vi "Setup Motors.vi"   [LabVIEW 2014]
uses:
  <vilib>/Rock Robotics/SystemInterfaces/DIO/FPGA_DIOPWMChannel.ctl
  <vilib>/Rock Robotics/WPI/Joystick/WPI_JoystickDeviceEnum.ctl
  <vilib>/Rock Robotics/SystemInterfaces/Typedef/FPGA_TypedefAnalogModule.ctl
  <vilib>/Rock Robotics/SystemInterfaces/AI/FPGA_AIChannel.ctl
  <vilib>/Rock Robotics/SystemInterfaces/Typedef/FPGA_TypedefDigitalModule.ctl
  <vilib>/Rock Robotics/WPI/Solenoid/WPI_SolenoidChannel.ctl
  <vilib>/Rock Robotics/SystemInterfaces/AI/FPGA_AIGyroChannel.ctl
  <vilib>/Rock Robotics/SystemInterfaces/Typedef/FPGA_TypedefAnalogModuleForGyro.ctl
  <vilib>/Rock Robotics/SystemInterfaces/DIO/FPGA_DIOChannel.ctl
  <vilib>/Rock Robotics/WPI/SafetyOutput/WPI_SafetyOutputConfigMenu.ctl
  NavX Code/navX-MXP Library/COMMON/TypeDefs/Value TypeDefs/navX Interface Protocol.ctl
  <vilib>/Rock Robotics/SystemInterfaces/spilib/spi_bus.ctl
  <vilib>/Rock Robotics/SystemInterfaces/i2clib/i2c_bus.ctl
  NavX Code/navX-MXP Library/COMMON/TypeDefs/Value TypeDefs/navX Update Rate.ctl
  <vilib>/Rock Robotics/WPI/MotorControl/WPI_MotorControlOpen Jaguar.vi
  <vilib>/Rock Robotics/WPI/MotorControl/WPI_MotorControlOpen Talon.vi
  <vilib>/Rock Robotics/WPI/Solenoid/WPI_SolenoidOpenSingle.vi
  <vilib>/Rock Robotics/WPI/Switch/WPI_SwitchOpenLimit.vi
  <vilib>/Rock Robotics/WPI/Counter/WPI_CounterDigitalInputToDigitalSource.vi
  <vilib>/Rock Robotics/WPI/Counter/WPI_CounterOpen UpDown Mode.vi
  Global Variables.vi
  NavX Code/navX-MXP Library/navX-MXP IMU.lvlib
types:
  T1 = typedef "navX-MXP IMU.lvlib/navX Update Rate.ctl" = u8
  T2 = typedef "i2c_bus.ctl" = enum16{"I2C On-Board", "I2C MXP", "Invalid"}
  T3 = typedef "spi_bus.ctl" = enum16{"SPI On-Board, CS0", "SPI On-Board, CS1", "SPI On-Board, CS2", "SPI On-Board, CS3", "SPI MXP", "Invalid"}
  T4 = typedef "navX-MXP IMU.lvlib/navX Interface Protocol.ctl" = enum16{"SPI", "I2C"}
  T5 = typedef "FPGA_DIOChannel.ctl" = enum8{"DIO 0", "DIO 1", "DIO 2", "DIO 3", "DIO 4", "DIO 5", "DIO 6", "DIO 7", "DIO 8", "DIO 9", "DIO MXP 0", "DIO MXP 1", "DIO MXP 2", "DIO MXP 3", "DIO MXP 4", "DIO MXP 5", "DIO MXP 6", "DIO MXP 7", "DIO MXP 8", "DIO MXP 9", "DIO MXP 10", "DIO MXP 11", "DIO MXP 12", "DIO MXP 13", "DIO MXP 14", "DIO MXP 15", "Invalid"}
  T6 = typedef "WPI_SafetyOutputConfigMenu.ctl" = enum16{"Enable", "Disable"}
  T7 = typedef "FPGA_TypedefDigitalModule.ctl" = enum16{"Controller 1"}
  T8 = typedef "FPGA_TypedefAnalogModuleForGyro.ctl" = enum16{"Controller 1"}
  T9 = typedef "FPGA_AIGyroChannel.ctl" = enum8{"AI 0", "AI 1", "Invalid"}
  T10 = typedef "WPI_SolenoidChannel.ctl" = enum8{"Solenoid 0", "Solenoid 1", "Solenoid 2", "Solenoid 3", "Solenoid 4", "Solenoid 5", "Solenoid 6", "Solenoid 7", "Invalid"}
  T11 = typedef "FPGA_DIOPWMChannel.ctl" = enum8{"PWM 0", "PWM 1", "PWM 2", "PWM 3", "PWM 4", "PWM 5", "PWM 6", "PWM 7", "PWM 8", "PWM 9", "PWM MXP 0", "PWM MXP 1", "PWM MXP 2", "PWM MXP 3", "PWM MXP 4", "PWM MXP 5", "PWM MXP 6", "PWM MXP 7", "PWM MXP 8", "PWM MXP 9", "Invalid"}
  T12 = typedef "FPGA_AIChannel.ctl" = enum8{"AI 0", "AI 1", "AI 2", "AI 3", "AI MXP 0", "AI MXP 1", "AI MXP 2", "AI MXP 3", "Invalid"}
  T13 = typedef "FPGA_TypedefAnalogModule.ctl" = enum16{"Controller 1"}
  T14 = typedef "WPI_JoystickDeviceEnum.ctl" = enum16{"USB 0", "USB 1", "USB 2", "USB 3", "USB 4", "USB 5"}
  T15 = typedef "WPI_MotorControlDeviceRef.ctl" = cluster{"DeviceStatus":errorcluster, "Type":T16, "PWM":cluster{"Controller":T7, "PWM Channel":T11, "DeadBand":T17}, "CAN":cluster{"Device Number":u8, "Control Mode":T18, "Semaphore":T19, "Max Vout":dbl, "TalonSRX Control Mode":T20}, "Invert":bool, "TransformRef":T21, "InvTransformRef":T21}
  T16 = typedef "WPI_MotorControlType.ctl" = enum16{"PWM", "CAN", "CANTalonSRX"}
  T17 = typedef "WPI_PWMDeadband.ctl" = cluster{"Name":string, "maxPositivePwm":i32, "minPositivePwm":i32, "centerPwm":i32, "maxNegativePwm":i32, "minNegativePwm":i32, "angularRange":u16}
  T18 = typedef "WPI_CANJaguar_ControlMode.ctl" = enum8{"Percent VBus", "Current", "Speed", "Position", "Voltage"}
  T19 = typedef "Semaphore RefNum" = refnum<k1>
  T20 = typedef "WPI_CANTalonSRX_APIControlMode.ctl" = enum8{"Percent VBus", "Speed", "Position", "Slave", "Unchanged / Invalid"}
  T21 = typedef "WPI_PWMTransform_ConPane.ctl" = refnum<vi>
  T22 = typedef "WPI_GyroDevRef.ctl" = cluster{"DevStatus":errorcluster, "Analog Module":T13, "Analog Channel":T12, "Offset":dbl, "Gain (VoltsPerDegree/Second)":dbl}
  T23 = typedef "WPI_SolenoidDevRef.ctl" = cluster{"DevStatus":errorcluster, "Pneumatics Control Module":u8, "Forward Solenoid Channel":T10, "Reverse Solenoid Channel":T10}
  T24 = typedef "WPI_SwitchDevRef.ctl" = cluster{"DevStatus":errorcluster, "DIO Channel":T5, "Controller":T7, "CntIndex":T25, "Normally Closed":bool}
  T25 = typedef "FPGA_CounterCtrSystemIndex.ctl" = enum8{"Ctr 0", "Ctr 1", "Ctr 2", "Ctr 3", "Ctr 4", "Ctr 5", "Ctr 6", "Ctr 7", "Invalid"}
  T26 = typedef "WPI_AnalogChannelDevRef.ctl" = cluster{"DevStatus":errorcluster, "Controller":T13, "Analog Channel":T12}
  T27 = typedef "WPI_DigitalInputDevRef.ctl" = cluster{"DevStatus":errorcluster, "DIO Channel":T5, "Controller":T7}
  T28 = typedef "FPGA_CounterEncoderSourceConvertionLVSourceType.ctl" = cluster{"DevStatus":errorcluster, "AnalogTriggerMode?":bool, "DigitalMode":cluster{"Controller":T7, "DIO Channel":T29}, "AnalogTriggerMode":cluster{"AnalogTriggerIndex":T30, "OutputType":T31}}
  T29 = typedef "FPGA_DIODigitalSourceChannel.ctl" = enum8{"DIO 0", "DIO 1", "DIO 2", "DIO 3", "DIO 4", "DIO 5", "DIO 6", "DIO 7", "DIO 8", "DIO 9", "DIO MXP 0", "DIO MXP 1", "DIO MXP 2", "DIO MXP 3", "DIO MXP 4", "DIO MXP 5", "DIO MXP 6", "DIO MXP 7", "DIO MXP 8", "DIO MXP 9", "DIO MXP 10", "DIO MXP 11", "DIO MXP 12", "DIO MXP 13", "DIO MXP 14", "DIO MXP 15", "Disabled"}
  T30 = typedef "FPGA_AnalogTriggerIndex.ctl" = enum8{"Trig 0", "Trig 1", "Trig 2", "Trig 3", "Trig 4", "Trig 5", "Trig 6", "Trig 7", "Invalid"}
  T31 = typedef "FPGA_AnalogTriggerOutType.ctl" = enum16{"InWindow", "TriggerState", "Rising", "Falling"}
  T32 = typedef "WPI_EncoderDevRef.ctl" = cluster{"DevStatus":errorcluster, "EncoderIndex":T33, "CounterIndex":T25, "DistancePerCount":dbl, "Decoding Type":T34}
  T33 = typedef "FPGA_EncoderIdx.ctl" = enum8{"Enc 0", "Enc 1", "Enc 2", "Enc 3", "Enc 4", "Enc 5", "Enc 6", "Enc 7", "Invalid"}
  T34 = typedef "WPI_EncoderType.ctl" = enum16{"1x", "2x", "4x"}
  T35 = typedef "WPI_CounterDevRef.ctl" = cluster{"DevStatus":errorcluster, "CntIndex":T25}
  T36 = typedef "navX-MXP IMU.lvlib/navX Device TypeDef.ctl" = cluster{"navX Interface Protocol":T4, "navX Interface Protocol TypeDefs":cluster{"SPIDevRef":T37, "I2CDevRef":T38}, "navX System Information":cluster{"Board Information":T39, "Status":T40, "Offsets":T44}, "navX Common Information":cluster{"Update Rate (4Hz-60Hz)":T1, "refnum name":string, "error":errorcluster}}
  T37 = typedef "WPI_SPIDevRef.ctl" = cluster{"DevStatus":errorcluster, "Handle":i32, "Controller":T7, "SPI Bus":T3}
  T38 = typedef "WPI_I2CDevRef.ctl" = cluster{"DevStatus":errorcluster, "Controller":T7, "Device Address":u8, "Handle":i32, "I2C Bus":T2}
  T39 = typedef "navX-MXP IMU.lvlib/navX Board Information.ctl" = cluster{"WhoAmI (50 | 0x32)":u8, "Board Revision":u8, "Firmware Major Version":u8, "Firmware Minor Version":u8}
  T40 = typedef "navX-MXP IMU.lvlib/navX Status Data.ctl" = cluster{"Update Rate Hz":u8, "Accelerometer Full-Scale Range":u8, "Gyro Full-Scale Range":u16, "NAVX_OP_STATUS":T41, "NAVX_CAL_STATUS":T42, "NAVX_SELFTEST_STATUS":u8, "NAVX_SENSOR_STATUS":T43}
  T41 = typedef "navX-MXP IMU.lvlib/navX NAVX_OP_STATUS.ctl" = u8
  T42 = typedef "navX-MXP IMU.lvlib/navX NAVX_CAL_STATUS.ctl" = u8
  T43 = typedef "navX-MXP IMU.lvlib/navX NAVX_SENSOR_STATUS.ctl" = cluster{"MOVING":bool, "YAW_STABLE":bool, "MAG_DISTURBANCE":bool, "ALTITUDE_VALID":bool, "SEALEVEL_PRESS_SET":bool, "FUSED_HEADING_VALID":bool}
  T44 = typedef "navX-MXP IMU.lvlib/navX Offsets Data.ctl" = cluster{"Yaw":dbl, "Quat W":dbl, "Quat X":dbl, "Quat Y":dbl, "Quat Z":dbl}
  T45 = typedef "WPI_JoystickDevRef.ctl" = cluster{"Device":T14}
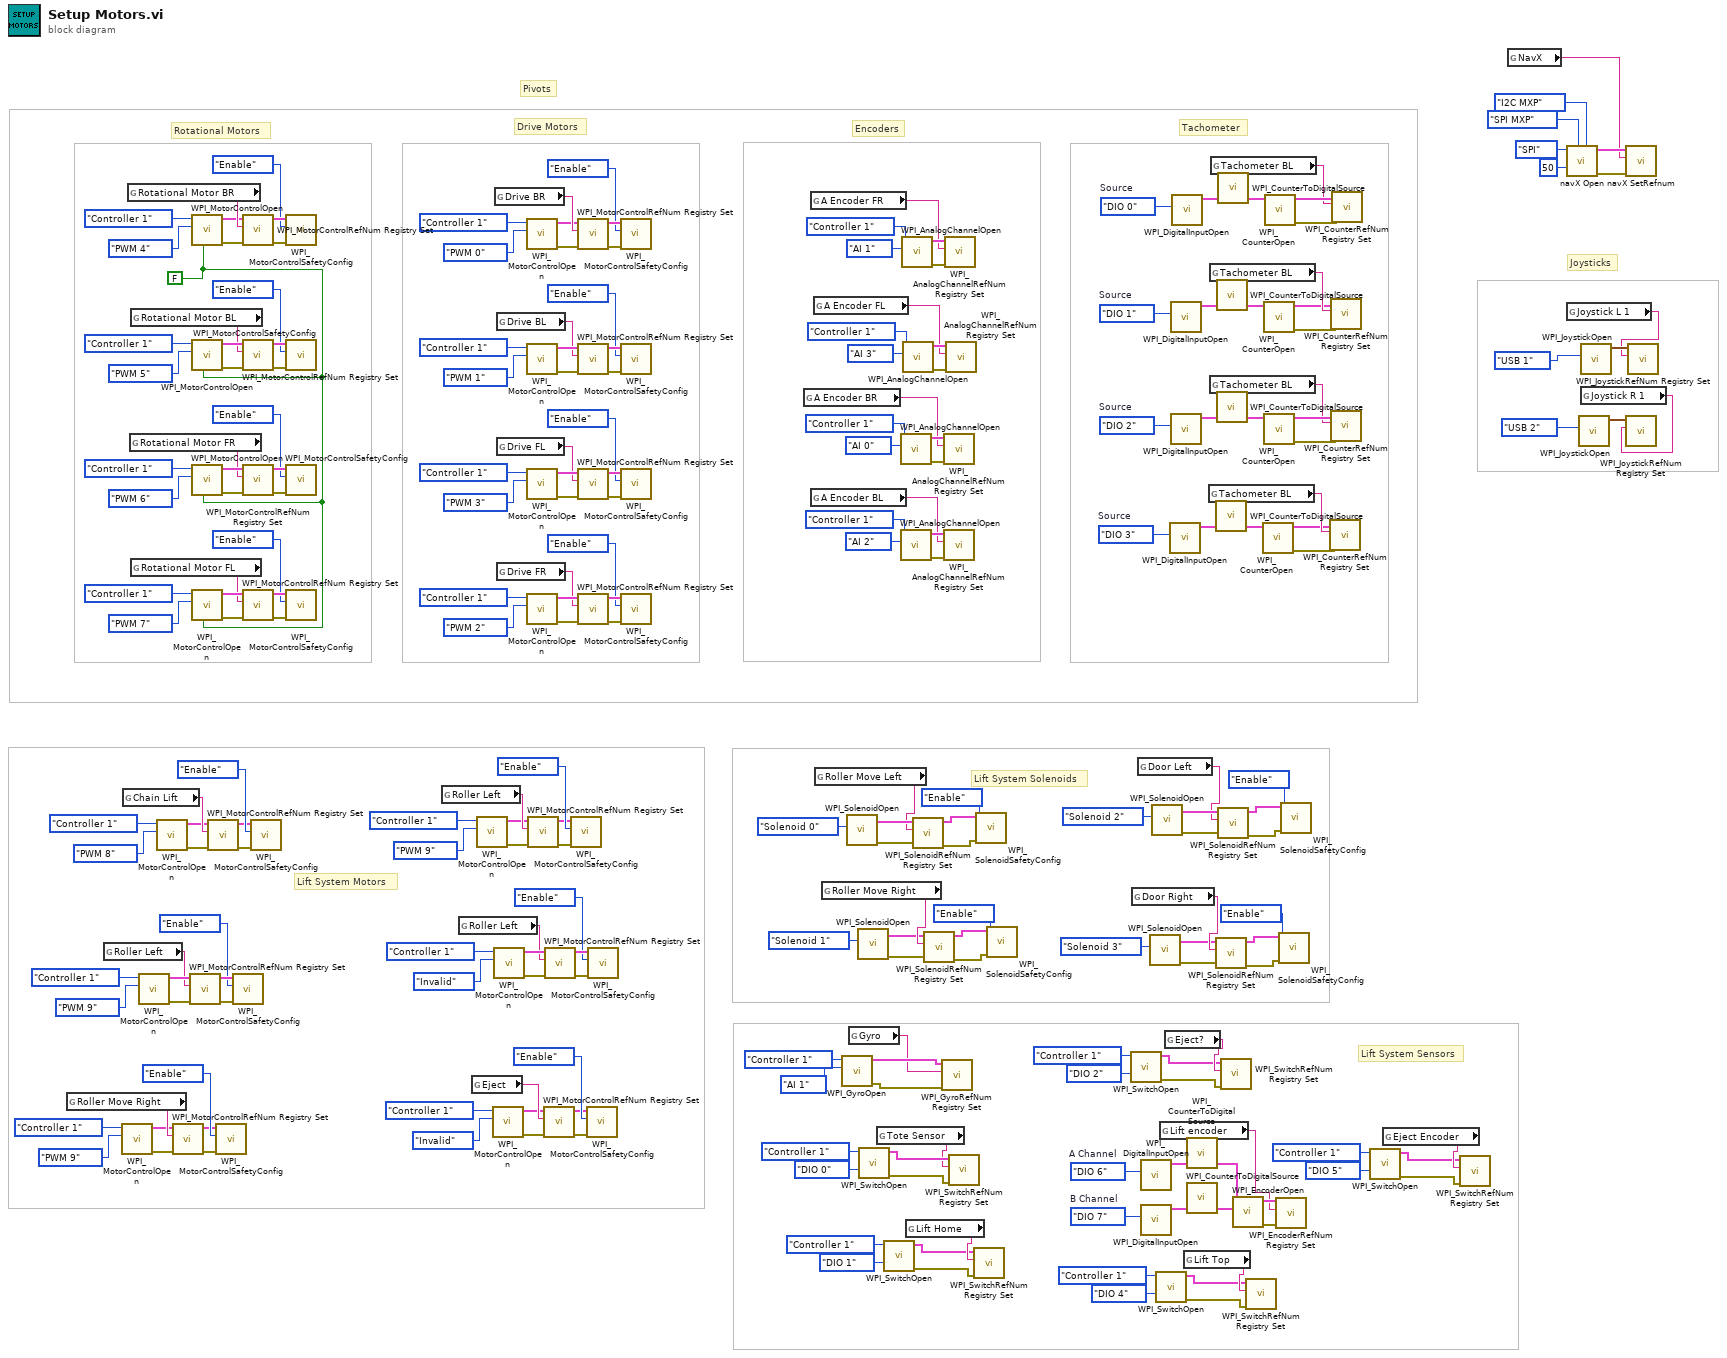
[diagram p0: block diagram]
diagram:
  w9 = FPGA_DIOChannel."DIO 3"  # Source
  w18 = FPGA_DIOChannel."DIO 2"  # Source
  w21 = FPGA_DIOChannel."DIO 1"  # Source
  w30 = FPGA_DIOChannel."DIO 0"  # Source
  w32 = FALSE ("Invert")
  w41 = FPGA_DIOChannel."DIO 7"  # B Channel
  w40 = FPGA_DIOChannel."DIO 6"  # A Channel
  # "Tachometer"
  # "Lift System Sensors"
  # "Lift System Solenoids"
  # "Lift System Motors"
  # "Encoders"
  # "Joysticks"
  # "Pivots"
  # "Rotational Motors"
  # "Drive Motors"
  n1 = global read "Global Variables.vi" "Roller Move Right"() -> (w130:string)
  n2 = global read "Global Variables.vi" "Roller Left"() -> (w133:string)
  n3 = call-poly <vilib>:"WPI_MotorControlOpen.vi"("PWM Channel"=FPGA_DIOPWMChannel."PWM 9", "Controller"=FPGA_TypedefDigitalModule."Controller 1") -> ("error out"=w125:errorcluster, "MotorControlDeviceRef"=w124:T15)  [unwired: 8 in]
  n4 = global read "Global Variables.vi" "Chain Lift"() -> (w146:string)
  n5 = global read "Global Variables.vi" "Rotational Motor BR"() -> (w200:string)
  n6 = global read "Global Variables.vi" "Rotational Motor FR"() -> (w174:string)
  n7 = global read "Global Variables.vi" "Rotational Motor BL"() -> (w175:string)
  n8 = global read "Global Variables.vi" "Rotational Motor FL"() -> (w173:string)
  n9 = call-poly <vilib>:"WPI_MotorControlOpen.vi"("PWM Channel"=FPGA_DIOPWMChannel."PWM 9", "Controller"=FPGA_TypedefDigitalModule."Controller 1") -> ("error out"=w138:errorcluster, "MotorControlDeviceRef"=w139:T15)  [unwired: 8 in]
  n10 = call-poly <vilib>:"WPI_MotorControlOpen.vi"("PWM Channel"=FPGA_DIOPWMChannel."PWM 8", "Controller"=FPGA_TypedefDigitalModule."Controller 1") -> ("error out"=w141:errorcluster, "MotorControlDeviceRef"=w140:T15)  [unwired: 8 in]
  n11 = call <vilib>:"WPI_MotorControlRefNum Registry Set.vi"("error in (no error)"=w125, "refnum name"=w130, "MotorControlDevRef"=w124) -> ("error out"=w127:errorcluster, "MotorControlDevRef"=w126:T15)  [unwired: 7 in]
  n12 = call <vilib>:"WPI_MotorControlRefNum Registry Set.vi"("error in (no error)"=w138, "refnum name"=w133, "MotorControlDevRef"=w139) -> ("error out"=w136:errorcluster, "MotorControlDevRef"=w137:T15)  [unwired: 7 in]
  n13 = call-poly <vilib>:"WPI_MotorControlOpen.vi"("Invert"=w32, "PWM Channel"=FPGA_DIOPWMChannel."PWM 4", "Controller"=FPGA_TypedefDigitalModule."Controller 1") -> ("error out"=w198:errorcluster, "MotorControlDeviceRef"=w199:T15)  [unwired: 7 in]
  n14 = call-poly <vilib>:"WPI_MotorControlOpen.vi"("Invert"=w32, "PWM Channel"=FPGA_DIOPWMChannel."PWM 5", "Controller"=FPGA_TypedefDigitalModule."Controller 1") -> ("error out"=w192:errorcluster, "MotorControlDeviceRef"=w193:T15)  [unwired: 7 in]
  n15 = call-poly <vilib>:"WPI_MotorControlOpen.vi"("Invert"=w32, "PWM Channel"=FPGA_DIOPWMChannel."PWM 6", "Controller"=FPGA_TypedefDigitalModule."Controller 1") -> ("error out"=w186:errorcluster, "MotorControlDeviceRef"=w187:T15)  [unwired: 7 in]
  n16 = call-poly <vilib>:"WPI_MotorControlOpen.vi"("Invert"=w32, "PWM Channel"=FPGA_DIOPWMChannel."PWM 7", "Controller"=FPGA_TypedefDigitalModule."Controller 1") -> ("error out"=w180:errorcluster, "MotorControlDeviceRef"=w181:T15)  [unwired: 7 in]
  n17 = call <vilib>:"WPI_MotorControlRefNum Registry Set.vi"("error in (no error)"=w141, "refnum name"=w146, "MotorControlDevRef"=w140) -> ("error out"=w143:errorcluster, "MotorControlDevRef"=w142:T15)  [unwired: 7 in]
  n18 = call <vilib>:"WPI_MotorControlSafetyConfig.vi"("error in (no error)"=w127, "mode"=WPI_SafetyOutputConfigMenu."Enable", "MotorControlDevRef"=w126) -> ()  [unwired: 7 in, 2 out]
  n19 = call <vilib>:"WPI_MotorControlSafetyConfig.vi"("error in (no error)"=w136, "mode"=WPI_SafetyOutputConfigMenu."Enable", "MotorControlDevRef"=w137) -> ()  [unwired: 7 in, 2 out]
  n20 = call <vilib>:"WPI_MotorControlRefNum Registry Set.vi"("error in (no error)"=w198, "refnum name"=w200, "MotorControlDevRef"=w199) -> ("error out"=w196:errorcluster, "MotorControlDevRef"=w197:T15)  [unwired: 7 in]
  n21 = call <vilib>:"WPI_MotorControlRefNum Registry Set.vi"("error in (no error)"=w192, "refnum name"=w175, "MotorControlDevRef"=w193) -> ("error out"=w190:errorcluster, "MotorControlDevRef"=w191:T15)  [unwired: 7 in]
  n22 = call <vilib>:"WPI_MotorControlRefNum Registry Set.vi"("error in (no error)"=w186, "refnum name"=w174, "MotorControlDevRef"=w187) -> ("error out"=w184:errorcluster, "MotorControlDevRef"=w185:T15)  [unwired: 7 in]
  n23 = call <vilib>:"WPI_MotorControlRefNum Registry Set.vi"("error in (no error)"=w180, "refnum name"=w173, "MotorControlDevRef"=w181) -> ("error out"=w178:errorcluster, "MotorControlDevRef"=w179:T15)  [unwired: 7 in]
  n24 = call <vilib>:"WPI_MotorControlSafetyConfig.vi"("error in (no error)"=w143, "mode"=WPI_SafetyOutputConfigMenu."Enable", "MotorControlDevRef"=w142) -> ()  [unwired: 7 in, 2 out]
  n25 = call <vilib>:"WPI_MotorControlSafetyConfig.vi"("error in (no error)"=w196, "mode"=WPI_SafetyOutputConfigMenu."Enable", "MotorControlDevRef"=w197) -> ()  [unwired: 7 in, 2 out]
  n26 = call <vilib>:"WPI_MotorControlSafetyConfig.vi"("error in (no error)"=w190, "mode"=WPI_SafetyOutputConfigMenu."Enable", "MotorControlDevRef"=w191) -> ()  [unwired: 7 in, 2 out]
  n27 = call <vilib>:"WPI_MotorControlSafetyConfig.vi"("error in (no error)"=w184, "mode"=WPI_SafetyOutputConfigMenu."Enable", "MotorControlDevRef"=w185) -> ()  [unwired: 7 in, 2 out]
  n28 = call <vilib>:"WPI_MotorControlSafetyConfig.vi"("error in (no error)"=w178, "mode"=WPI_SafetyOutputConfigMenu."Enable", "MotorControlDevRef"=w179) -> ()  [unwired: 7 in, 2 out]
  n29 = global read "Global Variables.vi" "Roller Left"() -> (w122:string)
  n30 = global read "Global Variables.vi" "Roller Left"() -> (w109:string)
  n31 = global read "Global Variables.vi" "Eject"() -> (w106:string)
  n32 = call-poly <vilib>:"WPI_MotorControlOpen.vi"("PWM Channel"=FPGA_DIOPWMChannel."PWM 9", "Controller"=FPGA_TypedefDigitalModule."Controller 1") -> ("error out"=w117:errorcluster, "MotorControlDeviceRef"=w116:T15)  [unwired: 8 in]
  n33 = call-poly <vilib>:"WPI_MotorControlOpen.vi"("PWM Channel"=FPGA_DIOPWMChannel."Invalid", "Controller"=FPGA_TypedefDigitalModule."Controller 1") -> ("error out"=w101:errorcluster, "MotorControlDeviceRef"=w100:T15)  [unwired: 8 in]
  n34 = call-poly <vilib>:"WPI_MotorControlOpen.vi"("PWM Channel"=FPGA_DIOPWMChannel."Invalid", "Controller"=FPGA_TypedefDigitalModule."Controller 1") -> ("error out"=w114:errorcluster, "MotorControlDeviceRef"=w115:T15)  [unwired: 8 in]
  n35 = global read "Global Variables.vi" "Drive BR"() -> (w237:string)
  n36 = global read "Global Variables.vi" "Drive BL"() -> (w212:string)
  n37 = global read "Global Variables.vi" "Drive FL"() -> (w211:string)
  n38 = global read "Global Variables.vi" "Drive FR"() -> (w210:string)
  n39 = call-poly <vilib>:"WPI_MotorControlOpen.vi"("PWM Channel"=FPGA_DIOPWMChannel."PWM 0", "Controller"=FPGA_TypedefDigitalModule."Controller 1") -> ("error out"=w235:errorcluster, "MotorControlDeviceRef"=w236:T15)  [unwired: 8 in]
  n40 = call-poly <vilib>:"WPI_MotorControlOpen.vi"("PWM Channel"=FPGA_DIOPWMChannel."PWM 1", "Controller"=FPGA_TypedefDigitalModule."Controller 1") -> ("error out"=w229:errorcluster, "MotorControlDeviceRef"=w230:T15)  [unwired: 8 in]
  n41 = call-poly <vilib>:"WPI_MotorControlOpen.vi"("PWM Channel"=FPGA_DIOPWMChannel."PWM 3", "Controller"=FPGA_TypedefDigitalModule."Controller 1") -> ("error out"=w223:errorcluster, "MotorControlDeviceRef"=w224:T15)  [unwired: 8 in]
  n42 = call-poly <vilib>:"WPI_MotorControlOpen.vi"("PWM Channel"=FPGA_DIOPWMChannel."PWM 2", "Controller"=FPGA_TypedefDigitalModule."Controller 1") -> ("error out"=w217:errorcluster, "MotorControlDeviceRef"=w218:T15)  [unwired: 8 in]
  n43 = call <vilib>:"WPI_MotorControlRefNum Registry Set.vi"("error in (no error)"=w117, "refnum name"=w122, "MotorControlDevRef"=w116) -> ("error out"=w119:errorcluster, "MotorControlDevRef"=w118:T15)  [unwired: 7 in]
  n44 = call <vilib>:"WPI_MotorControlRefNum Registry Set.vi"("error in (no error)"=w101, "refnum name"=w106, "MotorControlDevRef"=w100) -> ("error out"=w103:errorcluster, "MotorControlDevRef"=w102:T15)  [unwired: 7 in]
  n45 = call <vilib>:"WPI_MotorControlRefNum Registry Set.vi"("error in (no error)"=w114, "refnum name"=w109, "MotorControlDevRef"=w115) -> ("error out"=w112:errorcluster, "MotorControlDevRef"=w113:T15)  [unwired: 7 in]
  n46 = call <vilib>:"WPI_MotorControlSafetyConfig.vi"("error in (no error)"=w119, "mode"=WPI_SafetyOutputConfigMenu."Enable", "MotorControlDevRef"=w118) -> ()  [unwired: 7 in, 2 out]
  n47 = call <vilib>:"WPI_MotorControlRefNum Registry Set.vi"("error in (no error)"=w235, "refnum name"=w237, "MotorControlDevRef"=w236) -> ("error out"=w233:errorcluster, "MotorControlDevRef"=w234:T15)  [unwired: 7 in]
  n48 = call <vilib>:"WPI_MotorControlRefNum Registry Set.vi"("error in (no error)"=w229, "refnum name"=w212, "MotorControlDevRef"=w230) -> ("error out"=w227:errorcluster, "MotorControlDevRef"=w228:T15)  [unwired: 7 in]
  n49 = call <vilib>:"WPI_MotorControlRefNum Registry Set.vi"("error in (no error)"=w223, "refnum name"=w211, "MotorControlDevRef"=w224) -> ("error out"=w221:errorcluster, "MotorControlDevRef"=w222:T15)  [unwired: 7 in]
  n50 = call <vilib>:"WPI_MotorControlRefNum Registry Set.vi"("error in (no error)"=w217, "refnum name"=w210, "MotorControlDevRef"=w218) -> ("error out"=w215:errorcluster, "MotorControlDevRef"=w216:T15)  [unwired: 7 in]
  n51 = call <vilib>:"WPI_MotorControlSafetyConfig.vi"("error in (no error)"=w103, "mode"=WPI_SafetyOutputConfigMenu."Enable", "MotorControlDevRef"=w102) -> ()  [unwired: 7 in, 2 out]
  n52 = call <vilib>:"WPI_MotorControlSafetyConfig.vi"("error in (no error)"=w112, "mode"=WPI_SafetyOutputConfigMenu."Enable", "MotorControlDevRef"=w113) -> ()  [unwired: 7 in, 2 out]
  n53 = call <vilib>:"WPI_MotorControlSafetyConfig.vi"("error in (no error)"=w233, "mode"=WPI_SafetyOutputConfigMenu."Enable", "MotorControlDevRef"=w234) -> ()  [unwired: 7 in, 2 out]
  n54 = call <vilib>:"WPI_MotorControlSafetyConfig.vi"("error in (no error)"=w227, "mode"=WPI_SafetyOutputConfigMenu."Enable", "MotorControlDevRef"=w228) -> ()  [unwired: 7 in, 2 out]
  n55 = call <vilib>:"WPI_MotorControlSafetyConfig.vi"("error in (no error)"=w221, "mode"=WPI_SafetyOutputConfigMenu."Enable", "MotorControlDevRef"=w222) -> ()  [unwired: 7 in, 2 out]
  n56 = call <vilib>:"WPI_MotorControlSafetyConfig.vi"("error in (no error)"=w215, "mode"=WPI_SafetyOutputConfigMenu."Enable", "MotorControlDevRef"=w216) -> ()  [unwired: 7 in, 2 out]
  n57 = global read "Global Variables.vi" "A Encoder BR"() -> (w149:string)
  n58 = global read "Global Variables.vi" "A Encoder FR"() -> (w151:string)
  n59 = global read "Global Variables.vi" "A Encoder BL"() -> (w150:string)
  n60 = global read "Global Variables.vi" "A Encoder FL"() -> (w148:string)
  n61 = global read "Global Variables.vi" "Roller Move Left"() -> (w94:string)
  n62 = global read "Global Variables.vi" "Roller Move Right"() -> (w93:string)
  n63 = call <vilib>:"WPI_GyroOpen.vi"("Analog Channel"=FPGA_AIGyroChannel."AI 1", "Controller"=FPGA_TypedefAnalogModuleForGyro."Controller 1") -> ("error out"=w74:errorcluster, "GyroDevRef"=w75:T22)  [unwired: 7 in, 1 out]
  n64 = call-poly <vilib>:"WPI_SolenoidOpen.vi"("Solenoid Channel"=WPI_SolenoidChannel."Solenoid 0") -> ("error out"=w96:errorcluster, "SolenoidDevRef"=w97:T23)  [unwired: 9 in]
  n65 = global read "Global Variables.vi" "Gyro"() -> (w71:string)
  n66 = call-poly <vilib>:"WPI_SolenoidOpen.vi"("Solenoid Channel"=WPI_SolenoidChannel."Solenoid 1") -> ("error out"=w91:errorcluster, "SolenoidDevRef"=w90:T23)  [unwired: 9 in]
  n67 = call-poly <vilib>:"WPI_SwitchOpen.vi"("DIO Channel"=FPGA_DIOChannel."DIO 0", "Controller"=FPGA_TypedefDigitalModule."Controller 1") -> ("error out"=w69:errorcluster, "SwitchDevRef"=w70:T24)  [unwired: 8 in]
  n68 = global read "Global Variables.vi" "Tote Sensor"() -> (w66:string)
  n69 = call-poly <vilib>:"WPI_SwitchOpen.vi"("DIO Channel"=FPGA_DIOChannel."DIO 1", "Controller"=FPGA_TypedefDigitalModule."Controller 1") -> ("error out"=w62:errorcluster, "SwitchDevRef"=w61:T24)  [unwired: 8 in]
  n70 = call <vilib>:"WPI_AnalogChannelOpen.vi"("Analog Channel"=FPGA_AIChannel."AI 0", "Controller"=FPGA_TypedefAnalogModule."Controller 1") -> ("error out"=w158:errorcluster, "AIDeviceRef"=w159:T26)  [unwired: 8 in]
  n71 = call <vilib>:"WPI_AnalogChannelOpen.vi"("Analog Channel"=FPGA_AIChannel."AI 2", "Controller"=FPGA_TypedefAnalogModule."Controller 1") -> ("error out"=w154:errorcluster, "AIDeviceRef"=w155:T26)  [unwired: 8 in]
  n72 = call <vilib>:"WPI_AnalogChannelOpen.vi"("Analog Channel"=FPGA_AIChannel."AI 1", "Controller"=FPGA_TypedefAnalogModule."Controller 1") -> ("error out"=w166:errorcluster, "AIDeviceRef"=w167:T26)  [unwired: 8 in]
  n73 = call <vilib>:"WPI_AnalogChannelOpen.vi"("Analog Channel"=FPGA_AIChannel."AI 3", "Controller"=FPGA_TypedefAnalogModule."Controller 1") -> ("error out"=w162:errorcluster, "AIDeviceRef"=w163:T26)  [unwired: 8 in]
  n74 = global read "Global Variables.vi" "Lift Home"() -> (w65:string)
  n75 = call <vilib>:"WPI_SolenoidRefNum Registry Set.vi"("error in (no error)"=w96, "refnum name"=w94, "SolenoidDevRef"=w97) -> ("error out"=w98:errorcluster, "SolenoidDevRef"=w99:T23)  [unwired: 7 in]
  n76 = call <vilib>:"WPI_SolenoidRefNum Registry Set.vi"("error in (no error)"=w91, "refnum name"=w93, "SolenoidDevRef"=w90) -> ("error out"=w89:errorcluster, "SolenoidDevRef"=w88:T23)  [unwired: 7 in]
  n77 = call <vilib>:"WPI_GyroRefNum Registry Set.vi"("error in (no error)"=w74, "refnum name"=w71, "GyroDevRef"=w75) -> ()  [unwired: 7 in, 2 out]
  n78 = call <vilib>:"WPI_AnalogChannelRefNum Registry Set.vi"("error in (no error)"=w158, "refnum name"=w149, "AIDeviceRef"=w159) -> ()  [unwired: 7 in, 2 out]
  n79 = call <vilib>:"WPI_AnalogChannelRefNum Registry Set.vi"("error in (no error)"=w154, "refnum name"=w150, "AIDeviceRef"=w155) -> ()  [unwired: 7 in, 2 out]
  n80 = call <vilib>:"WPI_AnalogChannelRefNum Registry Set.vi"("error in (no error)"=w166, "refnum name"=w151, "AIDeviceRef"=w167) -> ()  [unwired: 7 in, 2 out]
  n81 = call <vilib>:"WPI_AnalogChannelRefNum Registry Set.vi"("error in (no error)"=w162, "refnum name"=w148, "AIDeviceRef"=w163) -> ()  [unwired: 7 in, 2 out]
  n82 = call <vilib>:"WPI_SwitchRefNum Registry Set.vi"("error in (no error)"=w69, "refnum name"=w66, "SwitchDevRef"=w70) -> ()  [unwired: 7 in, 2 out]
  n83 = call <vilib>:"WPI_SwitchRefNum Registry Set.vi"("error in (no error)"=w62, "refnum name"=w65, "SwitchDevRef"=w61) -> ()  [unwired: 7 in, 2 out]
  n84 = call <vilib>:"WPI_SolenoidSafetyConfig.vi"("error in (no error)"=w98, "mode"=WPI_SafetyOutputConfigMenu."Enable", "SolenoidDevRef"=w99) -> ()  [unwired: 7 in, 2 out]
  n85 = call <vilib>:"WPI_SolenoidSafetyConfig.vi"("error in (no error)"=w89, "mode"=WPI_SafetyOutputConfigMenu."Enable", "SolenoidDevRef"=w88) -> ()  [unwired: 7 in, 2 out]
  n86 = call-poly <vilib>:"WPI_SwitchOpen.vi"("DIO Channel"=FPGA_DIOChannel."DIO 2", "Controller"=FPGA_TypedefDigitalModule."Controller 1") -> ("error out"=w52:errorcluster, "SwitchDevRef"=w51:T24)  [unwired: 8 in]
  n87 = global read "Global Variables.vi" "Door Right"() -> (w81:string)
  n88 = global read "Global Variables.vi" "Door Left"() -> (w82:string)
  n89 = call <vilib>:"WPI_DigitalInputOpen.vi"("DIO Channel"=w40) -> ("DigitalInputDevRef"=w37:T27)  [unwired: 2 in, 8 out]
  n90 = call <vilib>:"WPI_DigitalInputOpen.vi"("DIO Channel"=w41) -> ("DigitalInputDevRef"=w38:T27)  [unwired: 2 in, 8 out]
  n91 = call-poly <vilib>:"WPI_SolenoidOpen.vi"("Solenoid Channel"=WPI_SolenoidChannel."Solenoid 3") -> ("error out"=w79:errorcluster, "SolenoidDevRef"=w78:T23)  [unwired: 9 in]
  n92 = call-poly <vilib>:"WPI_SolenoidOpen.vi"("Solenoid Channel"=WPI_SolenoidChannel."Solenoid 2") -> ("error out"=w84:errorcluster, "SolenoidDevRef"=w85:T23)  [unwired: 9 in]
  n93 = call-poly <vilib>:"WPI_SwitchOpen.vi"("DIO Channel"=FPGA_DIOChannel."DIO 4", "Controller"=FPGA_TypedefDigitalModule."Controller 1") -> ("error out"=w57:errorcluster, "SwitchDevRef"=w56:T24)  [unwired: 8 in]
  n94 = global read "Global Variables.vi" "Lift encoder"() -> (w33:string)
  n95 = global read "Global Variables.vi" "Eject?"() -> (w55:string)
  n96 = call <vilib>:"WPI_DigitalInputOpen.vi"("DIO Channel"=w9) -> ("DigitalInputDevRef"=w10:T27)  [unwired: 2 in, 8 out]
  n97 = call <vilib>:"WPI_DigitalInputOpen.vi"("DIO Channel"=w21) -> ("DigitalInputDevRef"=w22:T27)  [unwired: 2 in, 8 out]
  n98 = call <vilib>:"WPI_DigitalInputOpen.vi"("DIO Channel"=w18) -> ("DigitalInputDevRef"=w17:T27)  [unwired: 2 in, 8 out]
  n99 = call <vilib>:"WPI_DigitalInputOpen.vi"("DIO Channel"=w30) -> ("DigitalInputDevRef"=w29:T27)  [unwired: 2 in, 8 out]
  n100 = global read "Global Variables.vi" "Lift Top"() -> (w60:string)
  n101 = call-poly <vilib>:"WPI_CounterToDigitalSource.vi"("DigitalInputDevRef"=w37) -> ("Digital Source"=w36:T28)  [unwired: 6 out]
  n102 = call-poly <vilib>:"WPI_CounterToDigitalSource.vi"("DigitalInputDevRef"=w38) -> ("Digital Source"=w39:T28)  [unwired: 6 out]
  n103 = global read "Global Variables.vi" "Tachometer BL"() -> (w13:string)
  n104 = global read "Global Variables.vi" "Tachometer BL"() -> (w25:string)
  n105 = global read "Global Variables.vi" "Tachometer BL"() -> (w14:string)
  n106 = global read "Global Variables.vi" "Tachometer BL"() -> (w26:string)
  n107 = call-poly <vilib>:"WPI_CounterToDigitalSource.vi"("DigitalInputDevRef"=w10) -> ("Digital Source"=w8:T28)  [unwired: 6 out]
  n108 = call <vilib>:"WPI_SolenoidRefNum Registry Set.vi"("error in (no error)"=w79, "refnum name"=w81, "SolenoidDevRef"=w78) -> ("error out"=w77:errorcluster, "SolenoidDevRef"=w76:T23)  [unwired: 7 in]
  n109 = call-poly <vilib>:"WPI_CounterToDigitalSource.vi"("DigitalInputDevRef"=w22) -> ("Digital Source"=w20:T28)  [unwired: 6 out]
  n110 = call-poly <vilib>:"WPI_CounterToDigitalSource.vi"("DigitalInputDevRef"=w17) -> ("Digital Source"=w19:T28)  [unwired: 6 out]
  n111 = call-poly <vilib>:"WPI_CounterToDigitalSource.vi"("DigitalInputDevRef"=w29) -> ("Digital Source"=w31:T28)  [unwired: 6 out]
  n112 = call <vilib>:"WPI_SolenoidRefNum Registry Set.vi"("error in (no error)"=w84, "refnum name"=w82, "SolenoidDevRef"=w85) -> ("error out"=w86:errorcluster, "SolenoidDevRef"=w87:T23)  [unwired: 7 in]
  n113 = call <vilib>:"WPI_SwitchRefNum Registry Set.vi"("error in (no error)"=w52, "refnum name"=w55, "SwitchDevRef"=w51) -> ()  [unwired: 7 in, 2 out]
  n114 = call <vilib>:"WPI_EncoderOpen.vi"("BSource"=w39, "ASource"=w36) -> ("error out"=w35:errorcluster, "EncoderDevRef"=w34:T32)  [unwired: 6 in, 2 out]
  n115 = call <vilib>:"WPI_SwitchRefNum Registry Set.vi"("error in (no error)"=w57, "refnum name"=w60, "SwitchDevRef"=w56) -> ()  [unwired: 7 in, 2 out]
  n116 = call-poly <vilib>:"WPI_CounterOpen.vi"("Up Source"=w8) -> ("error out"=w12:errorcluster, "CounterDevRef"=w11:T35)  [unwired: 6 in, 3 out]
  n117 = call-poly <vilib>:"WPI_CounterOpen.vi"("Up Source"=w20) -> ("error out"=w24:errorcluster, "CounterDevRef"=w23:T35)  [unwired: 6 in, 3 out]
  n118 = call-poly <vilib>:"WPI_CounterOpen.vi"("Up Source"=w19) -> ("error out"=w15:errorcluster, "CounterDevRef"=w16:T35)  [unwired: 6 in, 3 out]
  n119 = call-poly <vilib>:"WPI_CounterOpen.vi"("Up Source"=w31) -> ("error out"=w27:errorcluster, "CounterDevRef"=w28:T35)  [unwired: 6 in, 3 out]
  n120 = call <vilib>:"WPI_EncoderRefNum Registry Set.vi"("error in (no error)"=w35, "refnum name"=w33, "EncoderDevRef"=w34) -> ()  [unwired: 7 in, 2 out]
  n121 = call <vilib>:"WPI_SolenoidSafetyConfig.vi"("error in (no error)"=w77, "mode"=WPI_SafetyOutputConfigMenu."Enable", "SolenoidDevRef"=w76) -> ()  [unwired: 7 in, 2 out]
  n122 = call <vilib>:"WPI_SolenoidSafetyConfig.vi"("error in (no error)"=w86, "mode"=WPI_SafetyOutputConfigMenu."Enable", "SolenoidDevRef"=w87) -> ()  [unwired: 7 in, 2 out]
  n123 = call <vilib>:"WPI_CounterRefNum Registry Set.vi"("error in (no error)"=w12, "refnum name"=w13, "CounterDevRef"=w11) -> ()  [unwired: 7 in, 2 out]
  n124 = call <vilib>:"WPI_CounterRefNum Registry Set.vi"("error in (no error)"=w24, "refnum name"=w25, "CounterDevRef"=w23) -> ()  [unwired: 7 in, 2 out]
  n125 = call <vilib>:"WPI_CounterRefNum Registry Set.vi"("error in (no error)"=w15, "refnum name"=w14, "CounterDevRef"=w16) -> ()  [unwired: 7 in, 2 out]
  n126 = call <vilib>:"WPI_CounterRefNum Registry Set.vi"("error in (no error)"=w27, "refnum name"=w26, "CounterDevRef"=w28) -> ()  [unwired: 7 in, 2 out]
  n127 = call-poly <vilib>:"WPI_SwitchOpen.vi"("DIO Channel"=FPGA_DIOChannel."DIO 5", "Controller"=FPGA_TypedefDigitalModule."Controller 1") -> ("error out"=w47:errorcluster, "SwitchDevRef"=w46:T24)  [unwired: 8 in]
  n128 = global read "Global Variables.vi" "Eject Encoder"() -> (w50:string)
  n129 = call <vilib>:"WPI_SwitchRefNum Registry Set.vi"("error in (no error)"=w47, "refnum name"=w50, "SwitchDevRef"=w46) -> ()  [unwired: 7 in, 2 out]
  n130 = global read "Global Variables.vi" "NavX"() -> (w1:string)
  n131 = call "navX Open.vi"("I2C Bus"=i2c_bus."I2C MXP", "SPI Bus"=spi_bus."SPI MXP", "Update Rate (4Hz-60Hz)"=T1 50, "navX Interface Protocol"=navX_Interface_Protocol."SPI") -> ("error out"=w3:errorcluster, "navX Device TypeDef"=w2:T36)  [unwired: 5 in, 1 out]
  n132 = global read "Global Variables.vi" "Joystick L 1"() -> (w204:string)
  n133 = call <vilib>:"WPI_JoystickOpen.vi"("JoystickDevice"=WPI_JoystickDeviceEnum."USB 2") -> ("JoystickDevRef"=w202:T45)  [unwired: 10 in]
  n134 = call <vilib>:"WPI_JoystickOpen.vi"("JoystickDevice"=WPI_JoystickDeviceEnum."USB 1") -> ("JoystickDevRef"=w205:T45)  [unwired: 10 in]
  n135 = global read "Global Variables.vi" "Joystick R 1"() -> (w201:string)
  n136 = call "navX SetRefnum.vi"("error in (no error)"=w3, "refnum name"=w1, "navX Device TypeDef"=w2) -> ()  [unwired: 7 in, 2 out]
  n137 = call <vilib>:"WPI_JoystickRefNum Registry Set.vi"("refnum name"=w201, "JoystickDevRef"=w202) -> ()  [unwired: 8 in, 2 out]
  n138 = call <vilib>:"WPI_JoystickRefNum Registry Set.vi"("refnum name"=w204, "JoystickDevRef"=w205) -> ()  [unwired: 8 in, 2 out]
